vi "MFCcapability.vi"(10 "Ch Description":T3={"Ch Name"="", "Type"="", "Function"=enum."Analogue Input", "Ch State"=enum."On", "Calibration type"="", "A"=0.0, "B"=0.0, "C"=0.0, "D"=0.0, "Comments"="", "Address"={"Main"=0, "Ch."=0, "Sub"=0, "Port Name"=""}, "String"="", "Duty"=65535} {"Duty" format="%016b"; "D" format="%#_5g"; "C" format="%#_5g"; "B" format="%#_5g"; "A" format="%#_5g"}, 11 "MFCdescriptionIn":T1 {"mDot" format="%_4g"; "Setpoint" format="%.2g"; "MFCcapability"."MaxMdot" format="%_4g"; "MFCcapability"."MinMdot" format="%_4g"}) -> (3 "MFCdescriptionOut":T1 {"mDot" format="%_4g"; "Setpoint" format="%.2g"; "MFCcapability"."MaxMdot" format="%_4g"; "MFCcapability"."MinMdot" format="%_4g"})   [LabVIEW 2021]
uses:
  ADAM Client/Sub VIs/ADAM Controls/Ch_description_ADAM.ctl
  ADAM Client/Sub VIs/ADAM Controls/Module_type_ADAM.ctl
  ADAM Client/Sub VIs/ADAM Controls/Function_ADAM.ctl
  ADAM Client/Sub VIs/ADAM Controls/Channel_State.ctl
  ADAM Client/Sub VIs/ADAM Controls/Calib_type_ADAM.ctl
  ADAM Client/Sub VIs/ADAM Controls/Address.ctl
  MFCdescription.ctl
  MFCcapability.ctl
panel:
  # "AalborgMFC calibration is Zero and Span:\nA is minimum recommended demand, %\nB is mass flow for 0% readout\n\nC is maximum recommended demand, % \nD is mass flow for 100% readout"
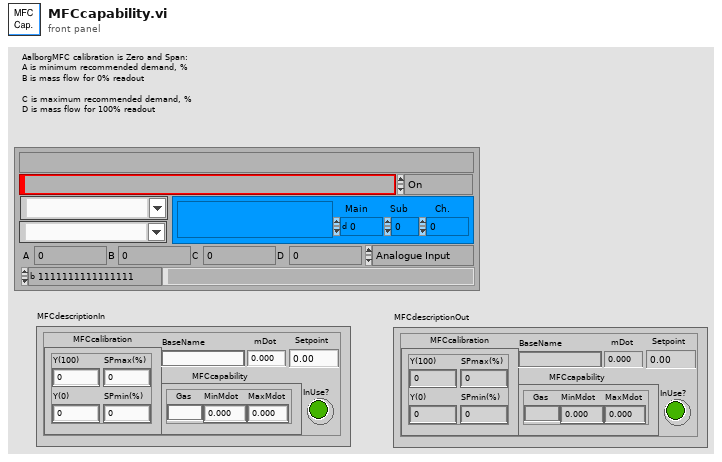
[diagram p1: front panel]
types:
  T1 = typedef "MFCdescription.ctl" = cluster{"BaseName":string, "MFCcalibration":cluster{"Y(100)":dbl, "Y(0)":dbl, "SPmin(%)":dbl, "SPmax(%)":dbl}, "MFCcapability":T2, "InUse?":bool, "Setpoint":dbl, "mDot":dbl}
  T2 = typedef "MFCcapability.ctl" = cluster{"Gas":string, "MinMdot":dbl, "MaxMdot":dbl}
  T3 = typedef "Ch_description_ADAM.ctl" = cluster{"Ch Name":string, "Type":T4, "Function":T5, "Ch State":T6, "Calibration type":T7, "A":dbl, "B":dbl, "C":dbl, "D":dbl, "Comments":string, "Address":T8, "String":string, "Duty":u16}
  T4 = typedef "Module_type_ADAM.ctl" = string
  T5 = typedef "Function_ADAM.ctl" = enum16{"Analogue Input", "Digital Input", "Event counter", "Event rate", "Analogue Output", "Digital Output", "Relay Output"}
  T6 = typedef "Channel_State.ctl" = enum16{"On", "Off", "Always On", "Always Off"}
  T7 = typedef "Calib_type_ADAM.ctl" = string
  T8 = typedef "Address.ctl" = cluster{"Main":i32, "Ch.":i32, "Sub":i32, "Port Name":string}
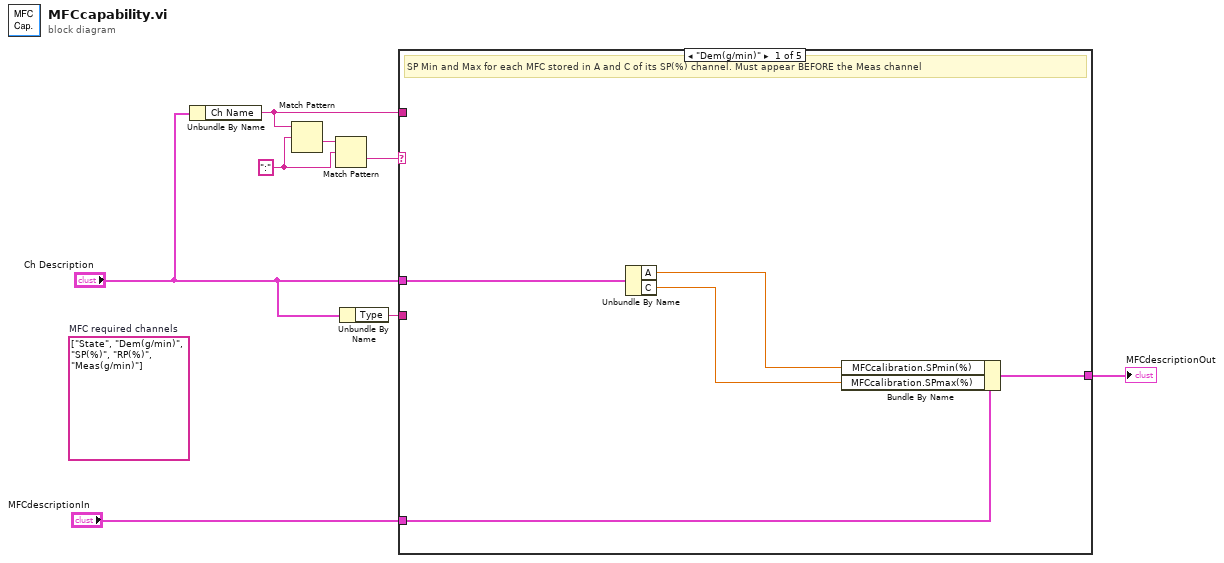
[diagram p0: block diagram]
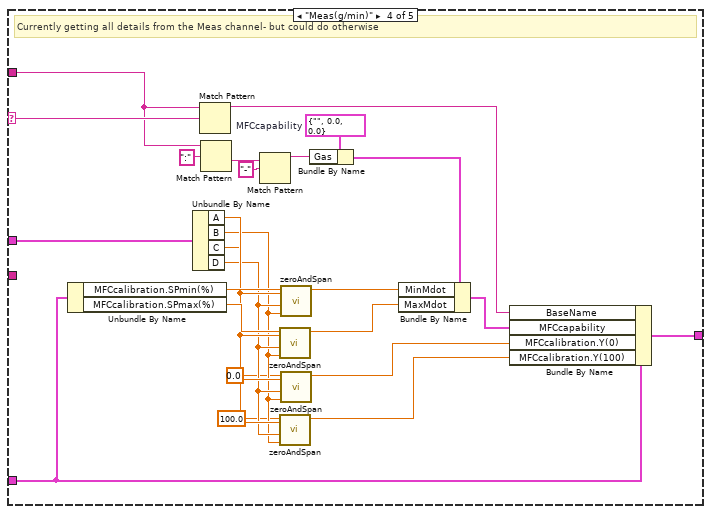
[diagram p4: hidden frame]
diagram:
  w4 = ":" ("regular expression")
  (unwired) string[] ["State", "Dem(g/min)", "SP(%)", "RP(%)", "Meas(g/min)"]  # MFC required channels
  n1 = Unbundle By Name("Ch Description") -> ("Ch Name"=w3:string)
  n2 = Match Pattern(string=w3, regular expression=w4) -> (after substring=w7:string)  [unwired: 1 in, 3 out]
  n3 = Match Pattern(string=w7, regular expression=w4) -> (after substring=w6:string)  [unwired: 1 in, 3 out]
  n4 = Unbundle By Name("Ch Description") -> ("Type"=w1:T4)
  n5 = case shown="\"Dem(g/min)\"" w6 {
    selector: w6 -> [_ _ _ w32 _]
    tunnel: [w13 w14 w15 w35 w41] -> w8
    tunnel: "Ch Description" -> [w12 _ _ w33 _]
    tunnel: "MFCdescriptionIn" -> [w11 w14 w15 w30 w41]
    tunnel: w3 -> [_ _ _ w16 _]
    tunnel: w1 -> [_ _ _ _ _]
    frame "Dem(g/min)" {
      # "SP Min and Max for each MFC stored in A and C of its SP(%) channel. Must appear BEFORE the Meas channel"
      n6 = Unbundle By Name(w12) -> ("A"=w10:dbl, "C"=w9:dbl)
      n7 = Bundle By Name(cluster=w11, "MFCcalibration.SPmin(%)"=w10, "MFCcalibration.SPmax(%)"=w9) -> (w13:T1)
    }
    frame "SP(%)" {
      # "SP Min and Max for each MFC stored in A and C of its SP(%) channel. Must appear BEFORE the Meas channel"
    }
    frame "RP(%)" {
    }
    frame "Meas(g/min)" {
      w40 = T2 {"Gas"="", "MinMdot"=0.0, "MaxMdot"=0.0}  # MFCcapability
      # "Currently getting all details from the Meas channel- but could do otherwise"
      n8 = Unbundle By Name(w30) -> ("MFCcalibration.SPmin(%)"=w28:dbl, "MFCcalibration.SPmax(%)"=w29:dbl)
      n9 = Unbundle By Name(w33) -> ("A"=w27:dbl, "B"=w24:dbl, "C"=w26:dbl, "D"=w25:dbl)
      n10 = Match Pattern(string=w16, regular expression=w32) -> (before substring=w31:string)  [unwired: 1 in, 3 out]
      n11 = Match Pattern(string=w16, regular expression=":") -> (after substring=w36:string)  [unwired: 1 in, 3 out]
      n12 = Match Pattern(string=w36, regular expression="-") -> (before substring=w37:string)  [unwired: 1 in, 3 out]
      n13 = call "zeroAndSpan.vi"("Xmax (100)"=w26, "Xmin (0)"=w27, "Ymin"=w24, "Ymax"=w25, "MeasuredX"=w29) -> ("calibratedY"=w17:dbl)  [unwired: 4 in, 2 out]
      n14 = call "zeroAndSpan.vi"("Xmax (100)"=w26, "Xmin (0)"=w27, "Ymin"=w24, "Ymax"=w25, "MeasuredX"=100.0) -> ("calibratedY"=w20:dbl)  [unwired: 4 in, 2 out]
      n15 = call "zeroAndSpan.vi"("Xmax (100)"=w26, "Xmin (0)"=w27, "Ymin"=w24, "Ymax"=w25, "MeasuredX"=w28) -> ("calibratedY"=w18:dbl)  [unwired: 4 in, 2 out]
      n16 = call "zeroAndSpan.vi"("Xmax (100)"=w26, "Xmin (0)"=w27, "Ymin"=w24, "Ymax"=w25, "MeasuredX"=0.0) -> ("calibratedY"=w21:dbl)  [unwired: 4 in, 2 out]
      n17 = Bundle By Name(cluster=w40, "Gas"=w37) -> (w34:T2)
      n18 = Bundle By Name(cluster=w34, "MinMdot"=w18, "MaxMdot"=w17) -> (w19:T2)
      n19 = Bundle By Name(cluster=w30, "BaseName"=w31, "MFCcapability"=w19, "MFCcalibration.Y(0)"=w21, "MFCcalibration.Y(100)"=w20) -> (w35:T1)
    }
    frame Default {
    }
  }
  "MFCdescriptionOut" <- w8
